vi "configure.vi"(8 "error in (no error)":errorcluster, 11 "DL090603DAQmxOnOffDetector in":refnum<class "DetectorDL090603DAQmxOnOff.lvclass">) -> (0 "error out":errorcluster, 3 "DL090603DAQmxOnOffDetector out":refnum<class "DetectorDL090603DAQmxOnOff.lvclass">)   [LabVIEW 2010, in "DetectorDL090603DAQmxOnOff.lvclass"]
uses:
  DetectorDL090603DAQmxOnOff.lvclass
  GenericDetector/GenericDetector/Type_enum.ctl
  common/xcontrols/XComponentSpecification/XComponentSpecification/XComponentSpecification.xctl
  DetectorDL090603DAQmxOnOff.lvclass/DetectorDL090603DAQmxOnOff.ctl
  common/classes/GenericComponent/GenericComponent/GenericComponent.lvclass
  GenericDetector/GenericDetector/GenericDetector.lvclass
panel:
  in  "digitalOut spec":T1(xcontrol)
  out "Configuration":string
  in  "Specify voltage?":bool
  out "LSID":string
  in  "Type":T2
  in  "SerialNumber":string
  in  "Model":string
  in  "Manufacturer":string
  in  "cancel button":bool
  in  "save button":bool
  # "Configure DL090603DAQmxOnOffDetector"
  # "DigitalOut component"
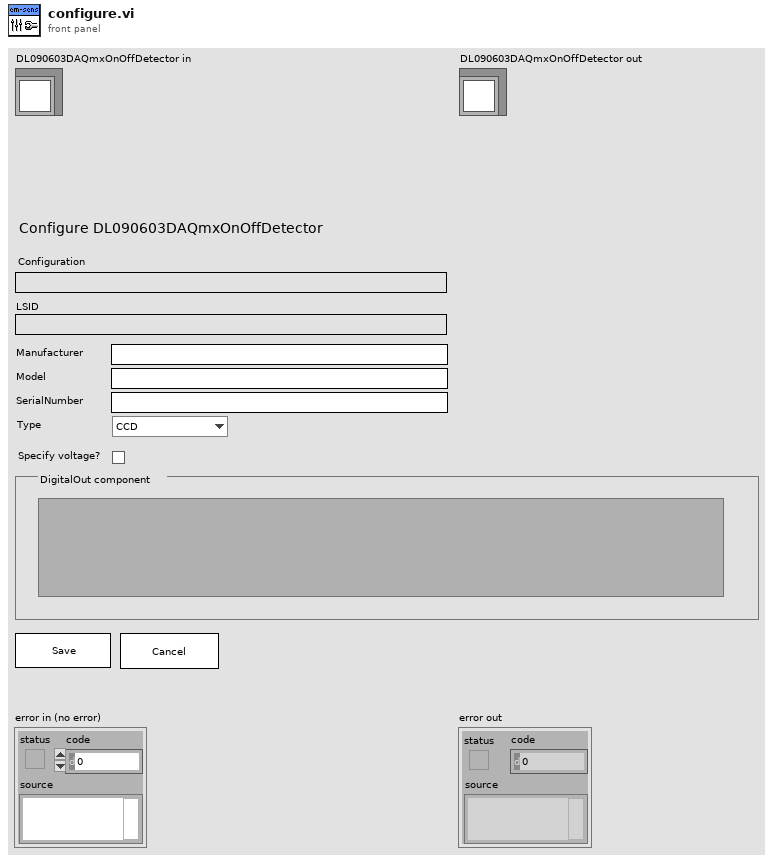
[diagram p1: front panel]
types:
  T1 = cluster{"class path":string, "configuration":string, "label":string, "settings name":string}
  T2 = typedef "GenericDetector.lvclass/type_enum.ctl" = enum16{"CCD", "IntensifiedCCD", "AnalogVideo", "PMT", "Photodiode", "Spectoscropy", "LifetimeImaging", "CorrelationSpectroscopy", "FTIR", "EM-CCD", "APD", "CMOS", "Unknown"}
  T3 = typedef "plugin_specification.ctl" = cluster{"class path":string, "configuration":string, "label":string, "settings name":string}
  T4 = typedef "LSID_cluster.ctl" = cluster{"identifier":string, "revision":i32}
  T5 = typedef "DetectorDL090603DAQmxOnOff.lvclass/config_data_cluster.ctl" = cluster{"DAQmxDigitalOut":T3, "manufacturer specification":T6, "type":T2, "LSID":T4, "specify voltage?":bool}
  T6 = typedef "manufacturer_specification_cluster.ctl" = cluster{"manufacturer":string, "model":string, "serial number":string, "lot number":string}
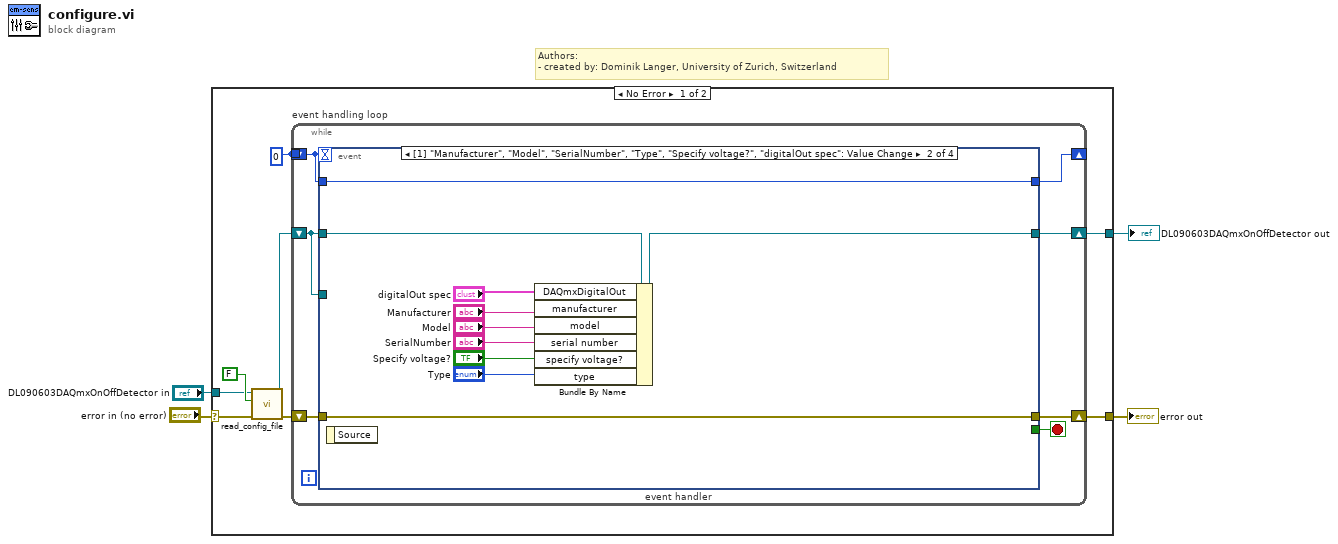
[diagram p0: block diagram]
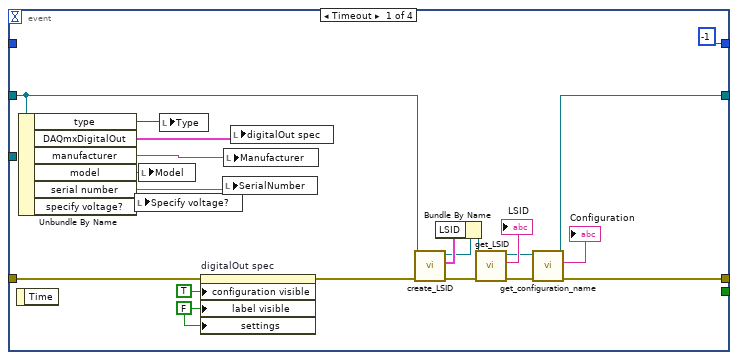
[diagram p2: hidden frame]
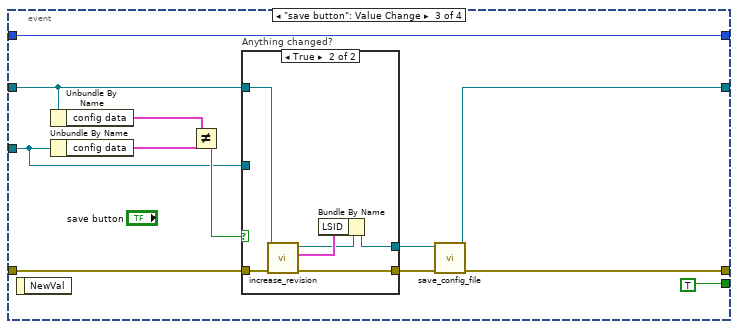
[diagram p3: hidden frame]
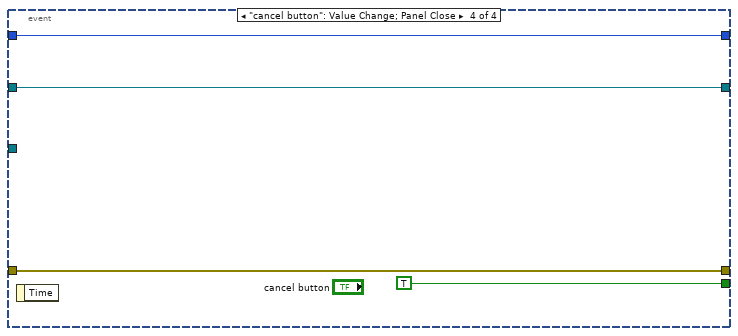
[diagram p5: hidden frame]
diagram:
  # "Authors: \n- created by: Dominik Langer, University of Zurich, Switzerland"
  n1 = case shown="No Error" "error in (no error)" {
    selector: "error in (no error)" -> [w7 w77]
    tunnel: [w12 w77] -> w2
    tunnel: [w11 w76] -> w1
    tunnel: "DL090603DAQmxOnOffDetector in" -> [w9 w76]
    frame No Error {
      w5 = 0
      n2 = call-dynamic "read_config_file.vi"("error in (no error)"=w7, "force load?"=FALSE, "GenericPlugin in"=w9) -> ("error out"=w6:errorcluster, "GenericPlugin out"=w8:refnum<class "DetectorDL090603DAQmxOnOff.lvclass">)  [unwired: 7 out]
      n3 = while "event handling loop" {
        shift-right: [w18] -> w12
        shift-left: w6 -> [w19]
        shift-right: [w17] -> w11
        shift-left: w8 -> [w13]
        shift-right: [w15] -> _
        shift-left: w5 -> [w16]
        tunnel: w5 -> [_]
        stop <- w14 stop-if-true
        n4 = event "event handler" shown="[1] \"Manufacturer\", \"Model\", \"SerialNumber\", \"Type\", \"Specify voltage?\", \"digitalOut spec\": Value Change" {
          selector: _ -> [_ _ _ _]
          dyn-events: _ -> [_ _ _ _]
          timeout: w16 -> [_ _ _ _]
          tunnel: w19 -> [w23 w45 w59 w75]
          tunnel: [w36 w45 w61 w75] -> w18
          tunnel: w13 -> [w34 w44 w56 w74]
          tunnel: [w28 w43 w60 w74] -> w17
          tunnel: w16 -> [_ w51 w63 w73]
          tunnel: [-1 w51 w63 w73] -> w15
          tunnel: [_ _ TRUE TRUE] -> w14
          tunnel: w13 -> [_ _ w53 _]
          event Timeout {
            w20 = FALSE ("label visible")
            n5 = event-data() -> ()  [unwired: 2 out]
            n6 = Unbundle By Name(w34) -> ("type"=w25:T2, "DAQmxDigitalOut"=w24:T3, "manufacturer"=w40:string, "model"=w39:string, "serial number"=w38:string, "specify voltage?"=w37:bool)
            n7 = local write "Specify voltage?"(w37) -> ()
            n8 = local write "Model"(w39) -> ()
            n9 = local write "Type"(w25) -> ()
            n10 = property on="digitalOut spec" class="XComponentSpecification (strict"(error in=w23, "configuration visible"=TRUE, "label visible"=w20, "settings"=w20) -> (error out=w22:errorcluster)  [unwired: 1 in, 1 out]
            n11 = local write "SerialNumber"(w38) -> ()
            n12 = local write "Manufacturer"(w40) -> ()
            n13 = local write "digitalOut spec"(w24) -> ()
            n14 = call-dynamic "create_LSID.vi"("error in (no error)"=w22, "GenericPlugin in"=w34) -> ("error out"=w33:errorcluster, "current LSID"=w31:T4, "GenericPlugin out"=w30:refnum<class "DetectorDL090603DAQmxOnOff.lvclass">)  [unwired: 7 in]
            n15 = Bundle By Name(cluster=w30, "LSID"=w31) -> (w29:refnum<class "DetectorDL090603DAQmxOnOff.lvclass">)
            n16 = call-dynamic "get_LSID.vi"("error in (no error)"=w33, "GenericPlugin in"=w29) -> ("error out"=w27:errorcluster, "LSID (string)"=→"LSID":string, "GenericPlugin out"=w26:refnum<class "DetectorDL090603DAQmxOnOff.lvclass">)  [unwired: 6 in, 1 out]
            n17 = call "get_configuration_name.vi"("error in (no error)"=w27, "GenericPlugin.lvclass in"=w26) -> ("error out"=w36:errorcluster, "configuration name"=→"Configuration":string, "GenericPlugin.lvclass out"=w28:refnum<class "DetectorDL090603DAQmxOnOff.lvclass">)  [unwired: 7 in]
          }
          event "Manufacturer", "Model", "SerialNumber", "Specify voltage?", "digitalOut spec": Value Change {
            n18 = event-data() -> ()  [unwired: 2 out]
            n19 = Bundle By Name(cluster=w44, "DAQmxDigitalOut"="digitalOut spec", "manufacturer"="Manufacturer", "model"="Model", "serial number"="SerialNumber", "specify voltage?"="Specify voltage?", "type"="Type") -> (w43:refnum<class "DetectorDL090603DAQmxOnOff.lvclass">)
          }
          event "save button": Value Change {
            n20 = event-data() -> ()  [unwired: 2 out]
            n21 = Unbundle By Name(w56) -> ("config data"=w54:T5)
            n22 = Unbundle By Name(w53) -> ("config data"=w55:T5)
            n23 = Not Equal?(x=w54, y=w55) -> (x != y?=w57:bool)
            n24 = case "Anything changed?" shown="True" w57 {
              tunnel: w59 -> [w65 w71]
              tunnel: [w65 w68] -> w58
              tunnel: w56 -> [_ w70]
              tunnel: [w64 w66] -> w52
              tunnel: w53 -> [w64 _]
              frame False {
              }
              frame True {
                n25 = call-dynamic "increase_revision.vi"("error in (no error)"=w71, "GenericPlugin in"=w70) -> ("error out"=w68:errorcluster, "new LSID"=w69:T4, "GenericPlugin out"=w67:refnum<class "DetectorDL090603DAQmxOnOff.lvclass">)  [unwired: 7 in]
                n26 = Bundle By Name(cluster=w67, "LSID"=w69) -> (w66:refnum<class "DetectorDL090603DAQmxOnOff.lvclass">)
              }
            }
            n27 = call-dynamic "save_config_file.vi"("error in (no error)"=w58, "GenericPlugin in"=w52) -> ("error out"=w61:errorcluster, "GenericPlugin out"=w60:refnum<class "DetectorDL090603DAQmxOnOff.lvclass">)  [unwired: 1 in, 7 out]
          }
          event "cancel button": Value Change; Panel Close {
            n28 = event-data() -> ()  [unwired: 2 out]
          }
        }
      }
    }
    frame Error {
    }
  }
  "error out" <- w2
  "DL090603DAQmxOnOffDetector out" <- w1
